vi "StringToBool_Ctl_2.vi"(10 "7 Bit word (str)":string) -> (1 "Bool Out":bool[](array[boolean]), 2 "Num Out":dbl[](array[numeric]))   [LabVIEW 2018]
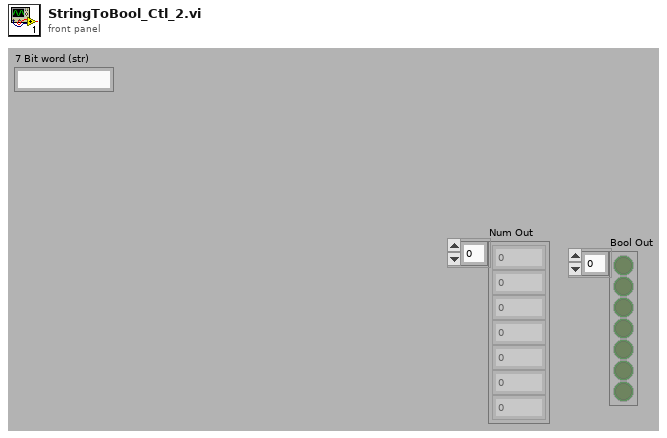
[diagram p1: front panel]
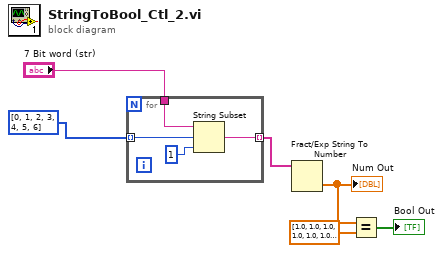
[diagram p0: block diagram]
diagram:
  n1 = for {
    tunnel: "7 Bit word (str)" -> [w10]
    tunnel: [w8] -> w4 mode=indexing
    tunnel: i32[] [0, 1, 2, 3, 4, 5, 6] -> [w7] mode=indexing
    n2 = String Subset(string=w10, offset (0)=w7, length (rest)=1 ("length (rest)")) -> (substring=w8:string)
  }
  n3 = Fract/Exp String To Number(string=w4) -> (number=w3:dbl[])  [unwired: 3 in, 1 out]
  "Num Out" <- w3
  n4 = Equal?(x=w3, y=dbl[] [1.0, 1.0, 1.0, 1.0, 1.0, 1.0, 1.0]) -> (x = y?=→"Bool Out":bool[])
